vi "Read Refs.vi"(11 "Attributes in":refnum<class "Attributes.lvclass">) -> (2 "Refs":refnum<class "Refs.lvclass">)   [LabVIEW 2025, in "jettl.lvlib" / "Attributes.lvclass"]
uses:
  Attributes.lvclass
  Refs/Refs.lvclass
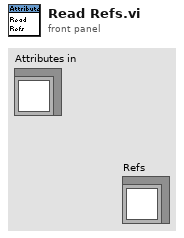
[diagram p1: front panel]
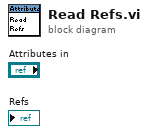
[diagram p0: block diagram]
diagram:
